vi "Teleop.vi"(10 "Match Info":T1={"Autonomous Elapsed Seconds"=0.0, "TeleOp Elapsed Seconds"=0.0, "Disabled Elapsed Seconds"=0.0, "Visited Autonomous"=FALSE, "Visited TeleOp"=FALSE, "Visited Disabled"=FALSE, "Autonomous Settings"={"Autonomous Style"=enum."Independent", "VI Refnum"=refnum}}, 11 "Call Context":T2) -> ()   [LabVIEW 2012]
doc: "This VI is called for each TeleOp packet received from the DS where the robot is not disabled. It is often used to read from the joysticks and update I/O or to update setpoints for timed control loops. It should complete and return within 20 milliseconds or it may miss DS packets."
uses:
  <vilib>/Rock Robotics/WPI/DriverStation/WPI_DriverStationDerivedRobotMode.ctl
  <vilib>/Rock Robotics/WPI/DriverStation/WPI_DriverStationMatch Info.ctl
  Begin/Robot Global Data.vi
  Begin/Global Refnums.vi
  Begin/Global Variables.vi
  <vilib>/Rock Robotics/WPI/Joystick/WPI_JoystickGetSetRefNum.vi
panel:
  out "Numeric 1":dbl(slide) scale=0.0..100.0
  out "Boolean 2":bool
  out "Boolean 1":bool
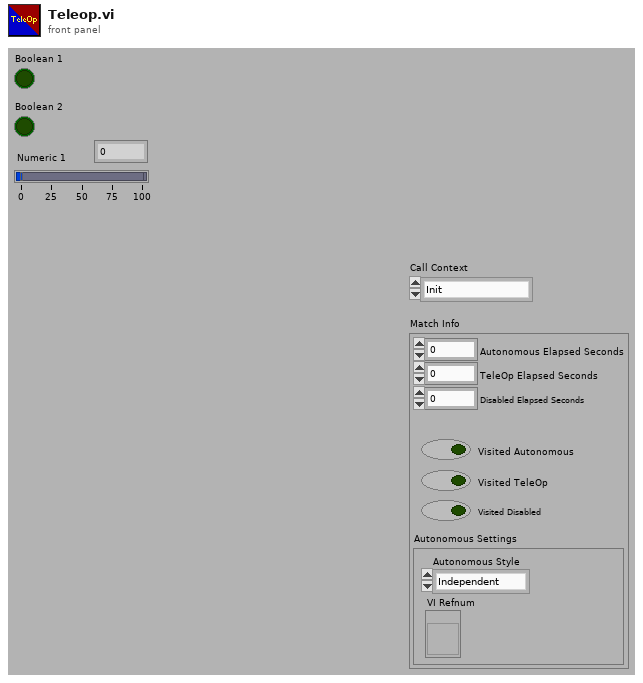
[diagram p1: front panel]
types:
  T1 = typedef "WPI_DriverStationMatch Info.ctl" = cluster{"Autonomous Elapsed Seconds":dbl, "TeleOp Elapsed Seconds":dbl, "Disabled Elapsed Seconds":dbl, "Visited Autonomous":bool, "Visited TeleOp":bool, "Visited Disabled":bool, "Autonomous Settings":cluster{"Autonomous Style":enum16{"Iterative", "Independent"}, "VI Refnum":refnum<vi>}}
  T2 = typedef "WPI_DriverStationDerivedRobotMode.ctl" = enum16{"Init", "Execute", "Stop"}
  T3 = typedef "WPI_JoystickDevRef.ctl" = cluster{"Device":T4}
  T4 = typedef "WPI_JoystickDeviceEnum.ctl" = enum16{"USB 1", "USB 2", "USB 3", "USB 4", "Kinect 1", "Kinect 2"}
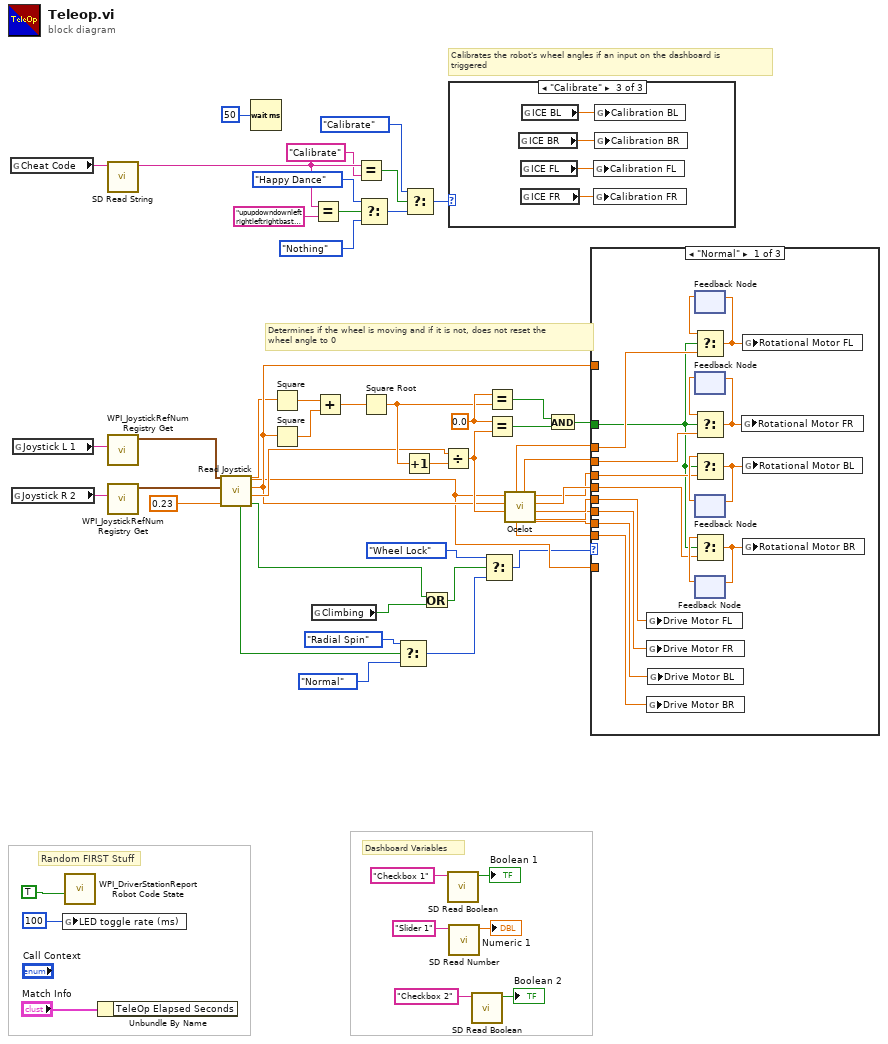
[diagram p0: block diagram]
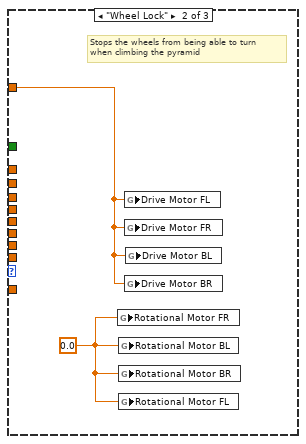
[diagram p2: hidden frame]
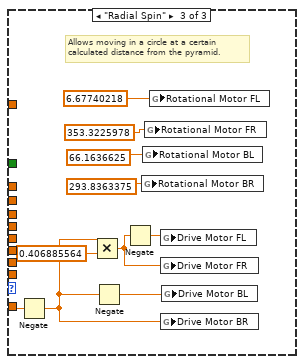
[diagram p3: hidden frame]
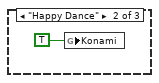
[diagram p5: hidden frame]
diagram:
  w29 = 0.0 ("x")
  # "Calibrates the robot's wheel angles if an input on the dashboard is \ntriggered"
  # "Determines if the wheel is moving and if it is not, does not reset the\nwheel angle to 0"
  # "Dashboard Variables"
  # "Random FIRST Stuff"
  n1 = global read "Global Refnums.vi" "Cheat Code"() -> (w46:string)
  n2 = global read "Global Refnums.vi" "Joystick R 2"() -> (w41:string)
  n3 = global read "Global Refnums.vi" "Joystick L 1"() -> (w42:string)
  n4 = global write "Robot Global Data.vi" "LED toggle rate (ms)"(u32 100 ("LED ms toggle rate")) -> ()
  n5 = call <vilib>:"WPI_DriverStationReport Robot Code State.vi"("TeleOp"=TRUE ("Autonomous")) -> ()  [unwired: 10 in, 1 out]
  n6 = Unbundle By Name("Match Info") -> ()  [unwired: 1 out]
  n7 = call <vilib>:"SD Read String.vi"("Name"=w46) -> ("String"=w47:string)  [unwired: 8 in, 2 out]
  n8 = call <vilib>:"WPI_JoystickRefNum Registry Get.vi"("refnum name"=w42) -> ("JoystickDevRef"=w43:T3)  [unwired: 9 in, 1 out]
  n9 = call <vilib>:"WPI_JoystickRefNum Registry Get.vi"("refnum name"=w41) -> ("JoystickDevRef"=w44:T3)  [unwired: 9 in, 1 out]
  n10 = call "Read Joystick.vi"("Joystick Deadbanded Value (default of 0.1)"=0.23, "Joystick R 2 DevRef"=w44, "Joystick L 1 DevRef"=w43) -> ("Wheel Lock"=w4:bool, "Joystick R 2 X Axis"=w7:dbl, "Joystick L 1 Y Axis"=w6:dbl, "Joystick L 1 X Axis"=w5:dbl, "Radial Spin"=w11:bool)  [unwired: 4 in]
  n11 = Wait (ms)(milliseconds to wait=u32 50) -> ()  [unwired: 1 out]
  n12 = Square(x=w5) -> (x^2=w35:dbl)
  n13 = Square(x=w6) -> (x^2=w36:dbl)
  n14 = global read "Global Variables.vi" "Climbing"() -> (w2:bool)
  n15 = Equal?(x=w47, y="upupdowndownleftrightleftrightbastart") -> (x = y?=w21:bool)
  n16 = Add(x=w35, y=w36) -> (x+y=w34:dbl)
  n17 = Equal?(x=w47, y="Calibrate") -> (x = y?=w25:bool)
  n18 = Select(t=enum16{"Nothing", "Happy Dance", "Calibrate"}."Happy Dance", s=w21, f=enum16{"Nothing", "Happy Dance", "Calibrate"}."Nothing") -> (s? t:f=w19:enum16{"Nothing", "Happy Dance", "Calibrate"})
  n19 = Square Root(x=w34) -> (sqrt(x)=w27:dbl)
  n20 = Select(t=enum16{"Normal", "Wheel Lock", "Radial Spin"}."Radial Spin", s=w11, f=enum16{"Normal", "Wheel Lock", "Radial Spin"}."Normal") -> (s? t:f=w12:enum16{"Normal", "Wheel Lock", "Radial Spin"})
  n21 = Increment(x=w27) -> (x+1=w28:dbl)
  n22 = Select(t=enum16{"Nothing", "Happy Dance", "Calibrate"}."Calibrate", s=w25, f=w19) -> (s? t:f=w23:enum16{"Nothing", "Happy Dance", "Calibrate"})
  n23 = Or(x=w4, y=w2) -> (x .or. y?=w3:bool)
  n24 = Divide(x=w7, y=w28) -> (x/y=w13:dbl)
  n25 = call <vilib>:"SD Read Boolean.vi"("Name"="Checkbox 1" ("refnum name")) -> ("Boolean"=→"Boolean 1":bool)  [unwired: 8 in, 2 out]
  n26 = case shown="\"Calibrate\"" w23 {
    frame "Nothing", Default {
    }
    frame "Happy Dance" {
      n27 = global write "Global Variables.vi" "Konami"(TRUE) -> ()
    }
    frame "Calibrate" {
      n28 = global read "Global Variables.vi" "ICE BR"() -> (w60:dbl)
      n29 = global read "Global Variables.vi" "ICE FL"() -> (w59:dbl)
      n30 = global read "Global Variables.vi" "ICE FR"() -> (w58:dbl)
      n31 = global read "Global Variables.vi" "ICE BL"() -> (w61:dbl)
      n32 = global write "Global Variables.vi" "Calibration FL"(w59) -> ()
      n33 = global write "Global Variables.vi" "Calibration FR"(w58) -> ()
      n34 = global write "Global Variables.vi" "Calibration BL"(w61) -> ()
      n35 = global write "Global Variables.vi" "Calibration BR"(w60) -> ()
    }
  }
  n36 = call <vilib>:"SD Read Number.vi"("Name"="Slider 1" ("refnum name")) -> ("Numeric"=→"Numeric 1":dbl)  [unwired: 8 in, 2 out]
  n37 = call <vilib>:"SD Read Boolean.vi"("Name"="Checkbox 2" ("refnum name")) -> ("Boolean"=→"Boolean 2":bool)  [unwired: 8 in, 2 out]
  n38 = Select(t=enum16{"Normal", "Wheel Lock", "Radial Spin"}."Wheel Lock", s=w3, f=w12) -> (s? t:f=w1:enum16{"Normal", "Wheel Lock", "Radial Spin"})
  n39 = Equal?(x=w29, y=w27) -> (x = y?=w31:bool)
  n40 = Equal?(x=w29, y=w13) -> (x = y?=w30:bool)
  n41 = call "Ocelot.vi"("RCW (X2)"=w13, "FWD (Y)"=w6, "STR (X)"=w5) -> ("FRD"=w16:dbl, "FLD"=w17:dbl, "BRS"=w39:dbl, "BLS"=w38:dbl, "BLD"=w15:dbl, "FRS"=w37:dbl, "BRD"=w14:dbl, "FLS"=w33:dbl)  [unwired: 1 in]
  n42 = And(x=w31, y=w30) -> (x .and. y?=w32:bool)
  n43 = case shown="\"Normal\"" w1 {
    tunnel: w39 -> [w74 _ _]
    tunnel: w38 -> [w73 _ _]
    tunnel: w37 -> [w72 _ _]
    tunnel: w33 -> [w69 _ _]
    tunnel: w32 -> [w66 _ _]
    tunnel: w17 -> [w65 _ _]
    tunnel: w16 -> [w64 _ _]
    tunnel: w15 -> [w63 _ _]
    tunnel: w14 -> [w62 _ _]
    tunnel: w5 -> [_ _ w85]
    tunnel: w6 -> [_ w79 _]
    frame "Normal" {
      n44 = global write "Global Variables.vi" "Drive Motor FL"(w65) -> ()
      n45 = global write "Global Variables.vi" "Drive Motor FR"(w64) -> ()
      n46 = global write "Global Variables.vi" "Drive Motor BR"(w62) -> ()
      n47 = global write "Global Variables.vi" "Drive Motor BL"(w63) -> ()
      n48 = feedback #1() -> (w78:dbl)  [unwired: 1 in]
      n49 = Select(t=w78, s=w66, f=w69) -> (s? t:f=w68:dbl)
      n50 = feedback-in #1(w68) -> ()
      n51 = feedback #2() -> (w77:dbl)  [unwired: 1 in]
      n52 = Select(t=w77, s=w66, f=w72) -> (s? t:f=w71:dbl)
      n53 = feedback-in #2(w71) -> ()
      n54 = feedback #3() -> (w76:dbl)  [unwired: 1 in]
      n55 = Select(t=w76, s=w66, f=w73) -> (s? t:f=w70:dbl)
      n56 = feedback-in #3(w70) -> ()
      n57 = feedback #4() -> (w75:dbl)  [unwired: 1 in]
      n58 = Select(t=w75, s=w66, f=w74) -> (s? t:f=w67:dbl)
      n59 = feedback-in #4(w67) -> ()
      n60 = global write "Global Variables.vi" "Rotational Motor FR"(w71) -> ()
      n61 = global write "Global Variables.vi" "Rotational Motor FL"(w68) -> ()
      n62 = global write "Global Variables.vi" "Rotational Motor BL"(w70) -> ()
      n63 = global write "Global Variables.vi" "Rotational Motor BR"(w67) -> ()
    }
    frame "Wheel Lock" {
      w80 = 0.0
      # "Stops the wheels from being able to turn\nwhen climbing the pyramid"
      n64 = global write "Global Variables.vi" "Rotational Motor FR"(w80) -> ()
      n65 = global write "Global Variables.vi" "Rotational Motor BL"(w80) -> ()
      n66 = global write "Global Variables.vi" "Rotational Motor BR"(w80) -> ()
      n67 = global write "Global Variables.vi" "Rotational Motor FL"(w80) -> ()
      n68 = global write "Global Variables.vi" "Drive Motor FL"(w79) -> ()
      n69 = global write "Global Variables.vi" "Drive Motor FR"(w79) -> ()
      n70 = global write "Global Variables.vi" "Drive Motor BR"(w79) -> ()
      n71 = global write "Global Variables.vi" "Drive Motor BL"(w79) -> ()
    }
    frame "Radial Spin" {
      # "Allows moving in a circle at a certain\ncalculated distance from the pyramid."
      n72 = Negate(x=w85) -> (-x=w81:dbl)
      n73 = Multiply(x=w81, y=0.406885564) -> (x*y=w84:dbl)
      n74 = Negate(x=w81) -> (-x=w82:dbl)
      n75 = Negate(x=w84) -> (-x=w83:dbl)
      n76 = global write "Global Variables.vi" "Rotational Motor BR"(293.8363375) -> ()
      n77 = global write "Global Variables.vi" "Rotational Motor BL"(66.1636625) -> ()
      n78 = global write "Global Variables.vi" "Rotational Motor FR"(353.3225978) -> ()
      n79 = global write "Global Variables.vi" "Rotational Motor FL"(6.67740218) -> ()
      n80 = global write "Global Variables.vi" "Drive Motor FL"(w83) -> ()
      n81 = global write "Global Variables.vi" "Drive Motor FR"(w84) -> ()
      n82 = global write "Global Variables.vi" "Drive Motor BR"(w81) -> ()
      n83 = global write "Global Variables.vi" "Drive Motor BL"(w82) -> ()
    }
  }
